vi "synch_mri_to_phys_data_vTriggerRunout.vi"() -> ()   [LabVIEW 2016]
uses:
  <vilib>/DAQmx/read.llb/DAQmx Read (Analog DBL 1Chan 1Samp).vi
  <vilib>/DAQmx/read.llb/DAQmx Read (Digital Bool 1Line 1Point).vi
  <vilib>/DAQmx/create/channels.llb/DAQmx Create Channel (DI-Digital Input).vi
  <vilib>/Instr/_visa.llb/VISA Configure Serial Port (Instr).vi
  <vilib>/DAQmx/create/channels.llb/DAQmx Create Channel (AI-Voltage-Basic).vi
  <vilib>/DAQmx/configure/timing.llb/DAQmx Timing (Sample Clock).vi
  <vilib>/DAQmx/miscellaneous.llb/DAQmx Fill In Error Info.vi
  <vilib>/Utility/file.llb/Write Delimited Spreadsheet (DBL).vi
panel:
  out "appended array":dbl[][](array[numeric])
  out "read buffer":string
  in  "stop":bool
  out "% SpO2":dbl[](graph)
  in  "SpO2 line":tag="MRITrig/ai0"
  out "Inspiration/Expiration":i16[](graph)
  out "Temp":dbl
  out "End":bool
  in  "TEST RUN":bool
  out "Temp (deg C)":dbl(slide) scale=0.0..40.0
  out "% CO_2":dbl format="%0.2f"
  out "% CO2":dbl[](graph)
  out "read byte count":u32=15
  out "write byte count":u32=8
  in  "\"Get Temperature\" command":string="\u0006ùGVT\u0001ð>"
  in  "file path (dialog if empty)":path=path "C:/Users/glihaug/Documents/Project 2/dc/dc171013_scan14_physdata.txt"
  in  "Sampling Rate":dbl=1000.0 format="%0.2f"
  in  "Mechanical Ventilator":tag="MRITrig/port0/line2"
  in  "CO2 line":tag="Dev0/ai1"
  in  "Dummy Ct":dbl=8.0
  out "Trigger Ct":dbl
  in  "COM Port":refnum<visa-resource-name>="COM5"
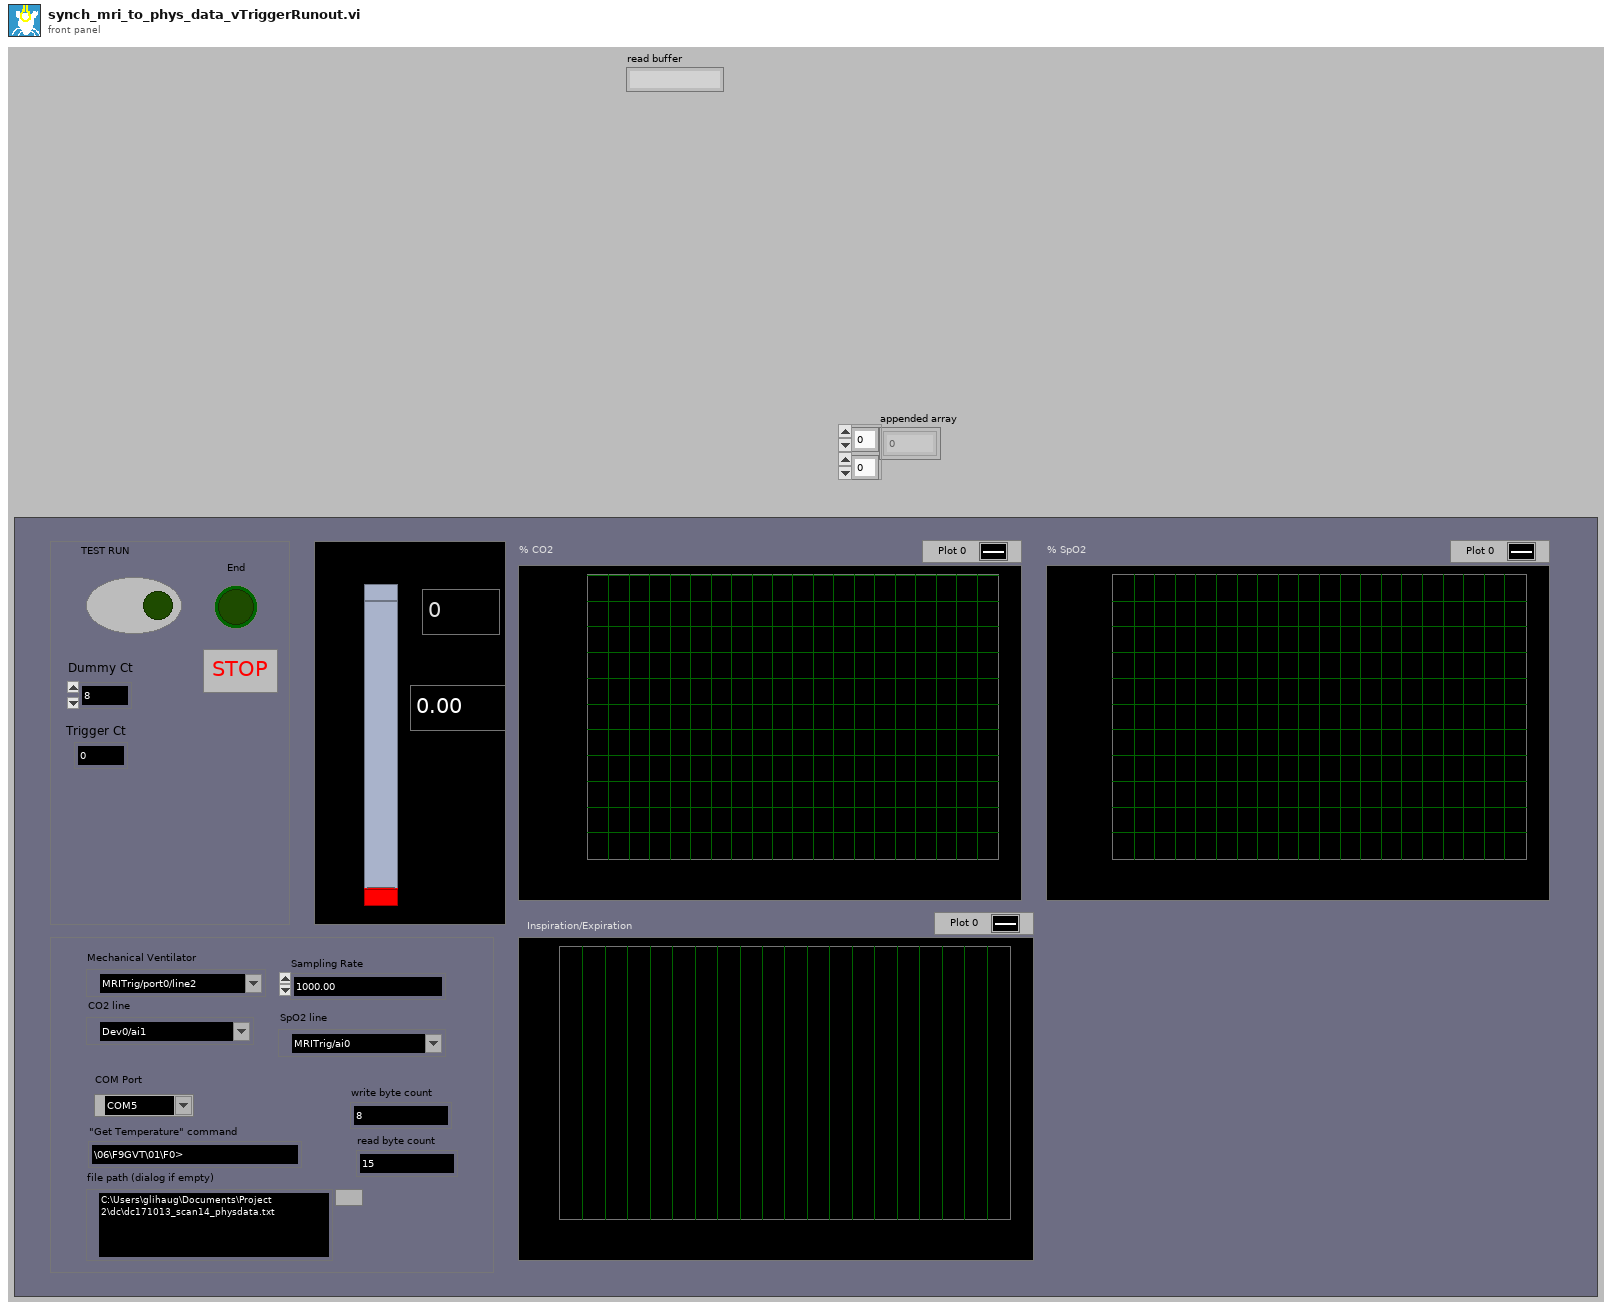
[diagram p1: front panel]
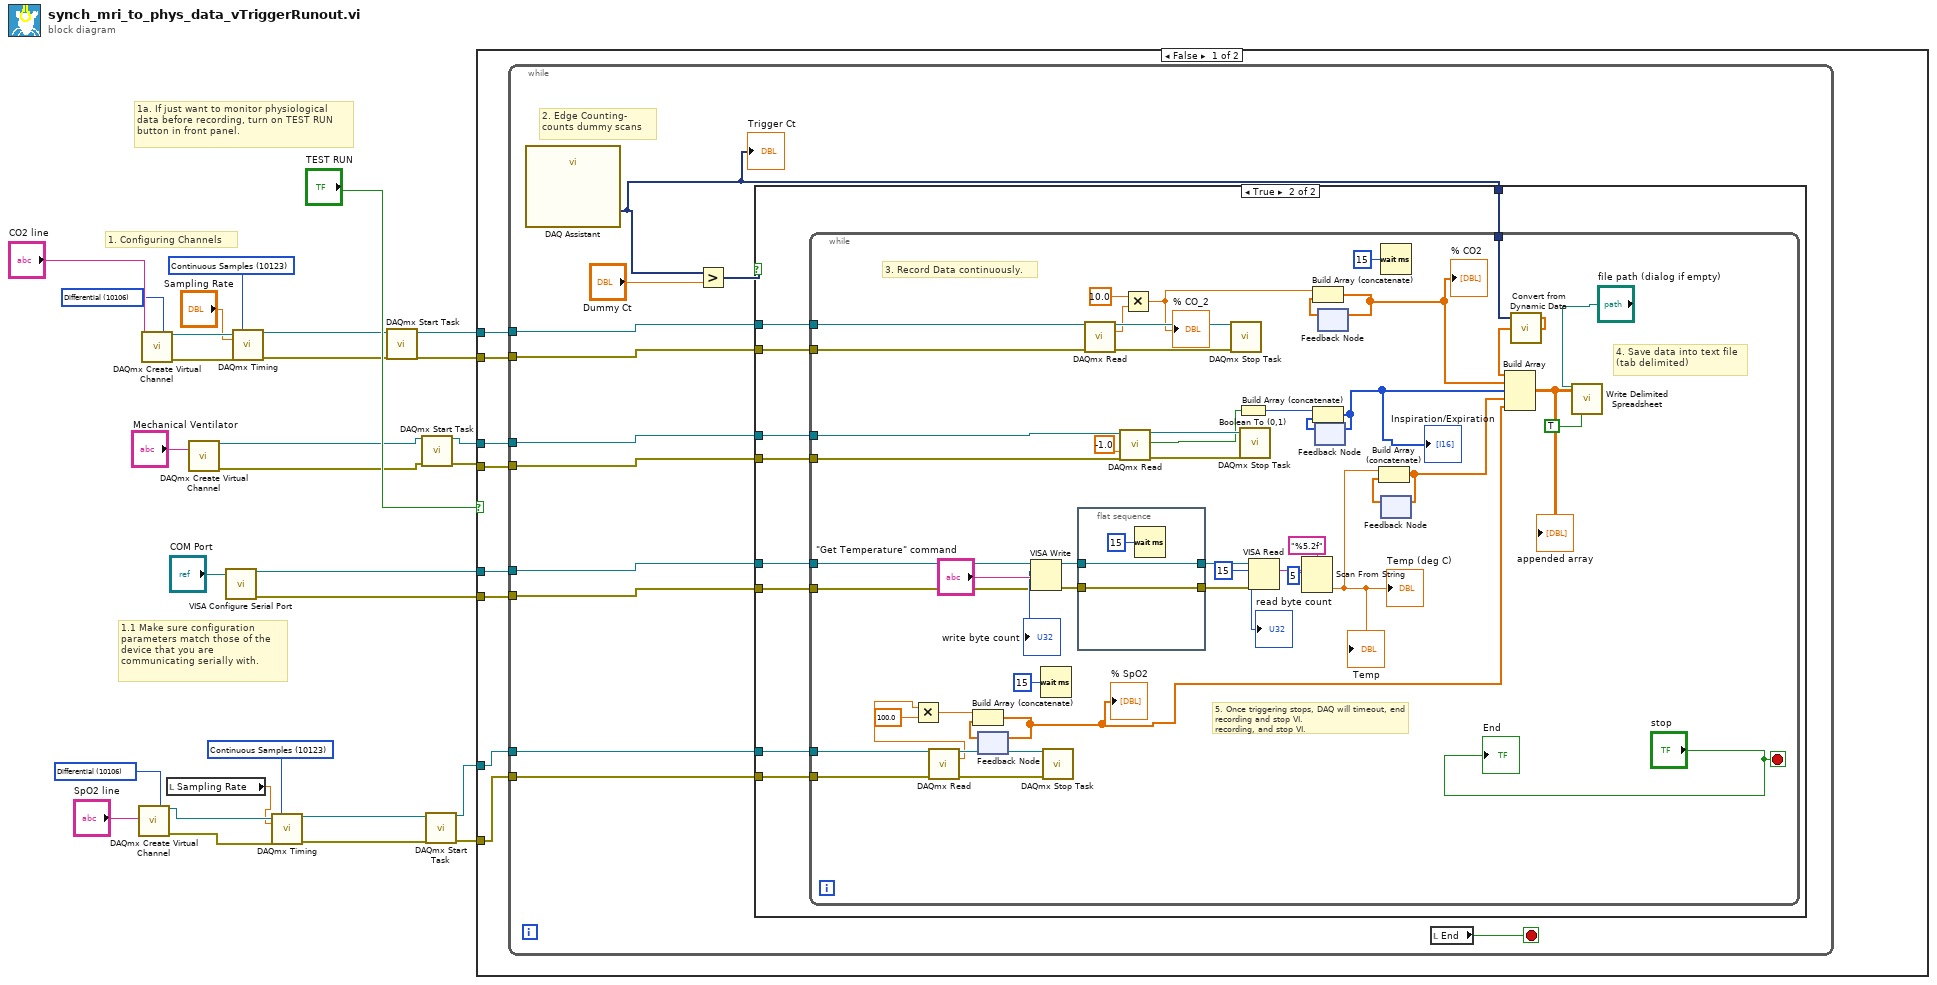
[diagram p0: block diagram]
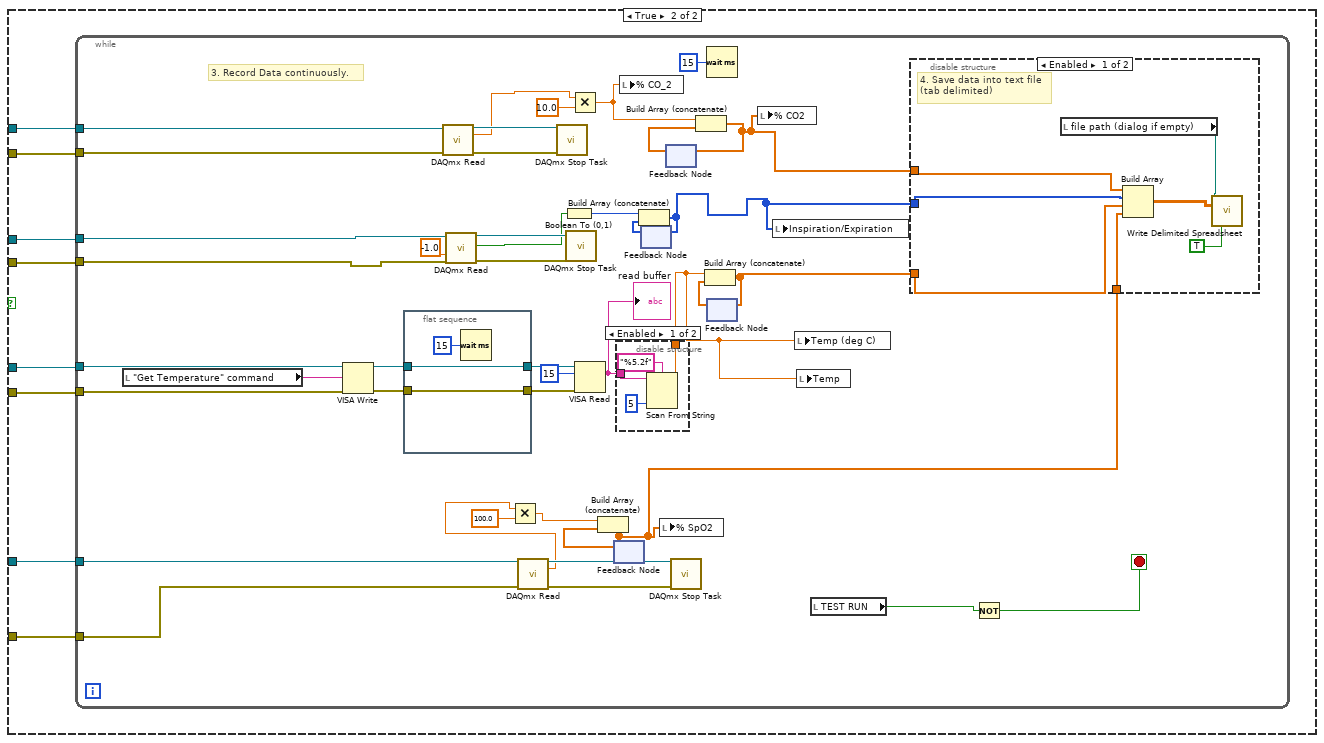
[diagram p3: hidden frame]
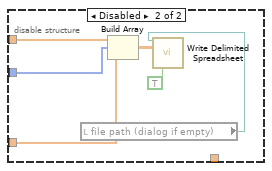
[diagram p5: hidden frame]
diagram:
  w8 = 10123 items=["Finite Samples"=10178, "Continuous Samples"=10123, "Hardware Timed Single Point"=12522] ("sample mode")
  w9 = 10106 items=["Default"=-1, "RSE"=10083, "NRSE"=10078, "Differential"=10106, "Pseudodifferential"=12529] ("input terminal configuration")
  w10 = 10106 items=["Default"=-1, "RSE"=10083, "NRSE"=10078, "Differential"=10106, "Pseudodifferential"=12529] ("input terminal configuration")
  w25 = 10123 items=["Finite Samples"=10178, "Continuous Samples"=10123, "Hardware Timed Single Point"=12522] ("sample mode")
  # "1a. If just want to monitor physiological\ndata before recording, turn on TEST RUN\nbutton in front panel."
  # "1.1 Make sure configuration\nparameters match those of the \ndevice that you are \ncommunicating serially with."
  # "1. Configuring Channels"
  n1 = call-poly <vilib>:"DAQmx Create Virtual Channel.vi"("input terminal configuration"=w9, "physical channels"="SpO2 line") -> ("task out"=w5:refnum<k21>, "error out"=w4:errorcluster)  [unwired: 12 in]
  n2 = call-poly <vilib>:"DAQmx Create Virtual Channel.vi"("input terminal configuration"=w10, "physical channels"="CO2 line") -> ("task out"=w28:refnum<k21>, "error out"=w27:errorcluster)  [unwired: 12 in]
  n3 = local read "Sampling Rate"() -> (w3:dbl)
  n4 = call-poly <vilib>:"DAQmx Create Virtual Channel.vi"("lines"="Mechanical Ventilator") -> ("task out"=w12:refnum<k21>, "error out"=w11:errorcluster)  [unwired: 13 in]
  n5 = call-poly "VISA Configure Serial Port"("VISA resource name"="COM Port") -> ("VISA resource name out"=w22:refnum<visa-resource-name>, "error out"=w21:errorcluster)  [unwired: 13 in]
  n6 = call-poly <vilib>:"DAQmx Timing.vi"("task/channels in"=w28, "sample mode"=w25, "rate"="Sampling Rate", "error in"=w27) -> ("task out"=w18:refnum<k21>, "error out"=w17:errorcluster)  [unwired: 10 in]
  n7 = call-poly <vilib>:"DAQmx Timing.vi"("task/channels in"=w5, "sample mode"=w8, "rate"=w3, "error in"=w4) -> ("task out"=w7:refnum<k21>, "error out"=w6:errorcluster)  [unwired: 10 in]
  n8 = call <vilib>:"DAQmx Start Task.vi"("task/channels in"=w18, "error in"=w17) -> ("task out"=w16:refnum<k21>, "error out"=w15:errorcluster)  [unwired: 12 in]
  n9 = call <vilib>:"DAQmx Start Task.vi"("task/channels in"=w12, "error in"=w11) -> ("task out"=w14:refnum<k21>, "error out"=w13:errorcluster)  [unwired: 12 in]
  n10 = call <vilib>:"DAQmx Start Task.vi"("task/channels in"=w7, "error in"=w6) -> ("task out"=w2:refnum<k21>, "error out"=w1:errorcluster)  [unwired: 12 in]
  n11 = case shown="False" "TEST RUN" {
    tunnel: w16 -> [w33 w116]
    tunnel: w15 -> [w32 w115]
    tunnel: w14 -> [w37 w120]
    tunnel: w13 -> [w36 w119]
    tunnel: w22 -> [w35 w118]
    tunnel: w21 -> [w34 w117]
    tunnel: w2 -> [w31 w114]
    tunnel: w1 -> [w30 w113]
    frame False {
      n12 = while {
        tunnel: w33 -> [w48]
        tunnel: w32 -> [w47]
        tunnel: w37 -> [w46]
        tunnel: w36 -> [w45]
        tunnel: w35 -> [w43]
        tunnel: w34 -> [w42]
        tunnel: w31 -> [w39]
        tunnel: w30 -> [w38]
        stop <- w44 stop-if-true
        # "2. Edge Counting-\ncounts dummy scans"
        n13 = call "DAQ Assistant"() -> ("data"=w40:dynamicdata)  [unwired: 16 in, 3 out]
        "Trigger Ct" <- w40
        n14 = Greater?(x=w40, y="Dummy Ct") -> (0:w49:dynamicdata)
        n15 = case shown="True" w49 {
          tunnel: w48 -> [_ w58]
          tunnel: w47 -> [_ w57]
          tunnel: w46 -> [_ w56]
          tunnel: w45 -> [_ w55]
          tunnel: w43 -> [_ w54]
          tunnel: w42 -> [_ w53]
          tunnel: w40 -> [_ w52]
          tunnel: w39 -> [_ w51]
          tunnel: w38 -> [_ w50]
          frame False {
          }
          frame True {
            n16 = while {
              tunnel: w58 -> [w77]
              tunnel: w57 -> [w76]
              tunnel: w56 -> [w75]
              tunnel: w55 -> [w74]
              tunnel: w54 -> [w95]
              tunnel: w53 -> [w94]
              tunnel: w52 -> [w73]
              tunnel: w51 -> [w63]
              tunnel: w50 -> [w62]
              stop <- "stop" stop-if-true
              # "5. Once triggering stops, DAQ will timeout, end recording and stop VI.\nrecording, and stop VI."
              # "4. Save data into text file \n(tab delimited)"
              # "3. Record Data continuously."
              n17 = call-poly <vilib>:"DAQmx Read.vi"("task/channels in"=w63, "error in"=w62) -> ("task out"=w67:refnum<k21>, "data"=w59:dbl, "error out"=w66:errorcluster)  [unwired: 11 in]
              n18 = Multiply(x=w59, y=100.0) -> (x*y=w60:dbl)
              n19 = feedback #1() -> (w64:dbl[])  [unwired: 1 in]
              n20 = Build Array (concatenate)(w60, w64) -> (w78:dbl[])
              "% SpO2" <- w78
              n21 = feedback-in #1(w78) -> ()
              n22 = VISA Write(VISA resource name=w95, write buffer="\"Get Temperature\" command", error in (no error)=w94) -> (VISA resource name out=w101:refnum<visa-resource-name>, return count=→"write byte count":u32, error out=w99:errorcluster)
              n23 = Wait (ms)(milliseconds to wait=u32 15) -> ()  [unwired: 1 out]
              n24 = call <vilib>:"DAQmx Stop Task.vi"("task/channels in"=w67, "error in"=w66) -> ()  [unwired: 12 in, 2 out]
              n25 = flat-sequence {
                tunnel: [w112] -> w100
                tunnel: w101 -> [w112]
                tunnel: w99 -> [w111]
                tunnel: [w111] -> w98
                frame #0 {
                  n26 = Wait (ms)(milliseconds to wait=u32 15) -> ()  [unwired: 1 out]
                }
              }
              n27 = call-poly <vilib>:"DAQmx Read.vi"("task/channels in"=w77, "error in"=w76) -> ("task out"=w106:refnum<k21>, "data"=w70:dbl, "error out"=w105:errorcluster)  [unwired: 11 in]
              n28 = call-poly <vilib>:"DAQmx Read.vi"("task/channels in"=w75, "timeout"=-1.0, "error in"=w74) -> ("task out"=w108:refnum<k21>, "data"=w93:bool, "error out"=w107:errorcluster)  [unwired: 10 in]
              n29 = Multiply(x=10.0, y=w70) -> (x*y=w68:dbl)
              "% CO_2" <- w68
              n30 = call <vilib>:"DAQmx Stop Task.vi"("task/channels in"=w106, "error in"=w105) -> ()  [unwired: 12 in, 2 out]
              n31 = Boolean To (0,1)(Boolean=w93) -> (0, 1=w90:i16)
              n32 = call <vilib>:"DAQmx Stop Task.vi"("task/channels in"=w108, "error in"=w107) -> ()  [unwired: 12 in, 2 out]
              n33 = VISA Read(VISA resource name=w100, byte count=u32 15, error in (no error)=w98) -> (read buffer=w83:string, return count=→"read byte count":u32)  [unwired: 2 out]
              n34 = Scan From String(format string="%5.2f", input string=w83, initial scan location=u32 5) -> (output 1=w82:dbl)  [unwired: 2 in, 3 out]
              "Temp (deg C)" <- w82
              "Temp" <- w82
              n35 = feedback #2() -> (w89:i16[])  [unwired: 1 in]
              n36 = Build Array (concatenate)(w90, w89) -> (w81:i16[])
              "Inspiration/Expiration" <- w81
              n37 = feedback-in #2(w81) -> ()
              n38 = feedback #3() -> (w92:dbl[])  [unwired: 1 in]
              n39 = Build Array (concatenate)(w68, w92) -> (w80:dbl[])
              "% CO2" <- w80
              n40 = feedback-in #3(w80) -> ()
              n41 = Wait (ms)(milliseconds to wait=u32 15) -> ()  [unwired: 1 out]
              n42 = feedback #4() -> (w88:dbl[])  [unwired: 1 in]
              n43 = Build Array (concatenate)(w82, w88) -> (w87:dbl[])
              n44 = feedback-in #4(w87) -> ()
              n45 = call "Convert from Dynamic Data"("Dynamic Data Type"=w73) -> ("Array"=w72:dbl[])  [unwired: 3 in]
              n46 = Build Array(w72, w80, w81, w87, w78) -> (w71:dbl[][])
              "appended array" <- w71
              n47 = call-poly <vilib>:"Write Delimited Spreadsheet.vi"("file path (dialog if empty)"="file path (dialog if empty)", "2D data"=w71, "transpose? (no:F)"=TRUE) -> ()  [unwired: 11 in, 2 out]
              "End" <- "stop"
            }
          }
        }
        n48 = local read "End"() -> (w44:bool)
      }
    }
    frame True {
      n49 = while {
        tunnel: w115 -> [w139]
        tunnel: w120 -> [w138]
        tunnel: w119 -> [w137]
        tunnel: w118 -> [w144]
        tunnel: w117 -> [w151]
        tunnel: w116 -> [w136]
        tunnel: w114 -> [w126]
        tunnel: w113 -> [w125]
        stop <- w141 stop-if-true
        # "3. Record Data continuously."
        n50 = local read "\"Get Temperature\" command"() -> (w143:string)
        n51 = VISA Write(VISA resource name=w144, write buffer=w143, error in (no error)=w151) -> (VISA resource name out=w155:refnum<visa-resource-name>, error out=w153:errorcluster)  [unwired: 1 out]
        n52 = flat-sequence {
          tunnel: [w182] -> w154
          tunnel: w155 -> [w182]
          tunnel: w153 -> [w181]
          tunnel: [w181] -> w152
          frame #0 {
            n53 = Wait (ms)(milliseconds to wait=u32 15) -> ()  [unwired: 1 out]
          }
        }
        n54 = call-poly <vilib>:"DAQmx Read.vi"("task/channels in"=w136, "error in"=w139) -> ("task out"=w159:refnum<k21>, "data"=w133:dbl, "error out"=w158:errorcluster)  [unwired: 11 in]
        n55 = call-poly <vilib>:"DAQmx Read.vi"("task/channels in"=w138, "timeout"=-1.0, "error in"=w137) -> ("task out"=w161:refnum<k21>, "data"=w150:bool, "error out"=w160:errorcluster)  [unwired: 10 in]
        n56 = call-poly <vilib>:"DAQmx Read.vi"("task/channels in"=w126, "error in"=w125) -> ("task out"=w129:refnum<k21>, "data"=w122:dbl, "error out"=w128:errorcluster)  [unwired: 11 in]
        n57 = Multiply(x=w122, y=100.0) -> (x*y=w123:dbl)
        n58 = call <vilib>:"DAQmx Stop Task.vi"("task/channels in"=w159, "error in"=w158) -> ()  [unwired: 12 in, 2 out]
        n59 = Boolean To (0,1)(Boolean=w150) -> (0, 1=w149:i16)
        n60 = call <vilib>:"DAQmx Stop Task.vi"("task/channels in"=w161, "error in"=w160) -> ()  [unwired: 12 in, 2 out]
        n61 = Multiply(x=w133, y=10.0) -> (x*y=w132:dbl)
        n62 = VISA Read(VISA resource name=w154, byte count=u32 15, error in (no error)=w152) -> (read buffer=w145:string)  [unwired: 3 out]
        "read buffer" <- w145
        n63 = feedback #5() -> (w127:dbl[])  [unwired: 1 in]
        n64 = Build Array (concatenate)(w123, w127) -> (w121:dbl[])
        n65 = feedback-in #5(w121) -> ()
        n66 = disable-structure shown="Enabled" {
          disable-tunnel: w145 -> [w164 _]
          disable-tunnel: [w163 _] -> w140
          frame Enabled {
            n67 = Scan From String(format string="%5.2f", input string=w164, initial scan location=u32 5) -> (output 1=w163:dbl)  [unwired: 2 in, 3 out]
          }
          frame Disabled {
          }
        }
        n68 = local write "% CO_2"(w132) -> ()
        n69 = feedback #6() -> (w148:i16[])  [unwired: 1 in]
        n70 = Build Array (concatenate)(w149, w148) -> (w135:i16[])
        n71 = feedback-in #6(w135) -> ()
        n72 = local write "% SpO2"(w121) -> ()
        n73 = feedback #7() -> (w131:dbl[])  [unwired: 1 in]
        n74 = call <vilib>:"DAQmx Stop Task.vi"("task/channels in"=w129, "error in"=w128) -> ()  [unwired: 12 in, 2 out]
        n75 = Build Array (concatenate)(w132, w131) -> (w130:dbl[])
        n76 = feedback-in #7(w130) -> ()
        n77 = Wait (ms)(milliseconds to wait=u32 15) -> ()  [unwired: 1 out]
        n78 = feedback #8() -> (w147:dbl[])  [unwired: 1 in]
        n79 = Build Array (concatenate)(w140, w147) -> (w146:dbl[])
        n80 = feedback-in #8(w146) -> ()
        n81 = local write "% CO2"(w130) -> ()
        n82 = local write "Inspiration/Expiration"(w135) -> ()
        n83 = local write "Temp (deg C)"(w140) -> ()
        n84 = local write "Temp"(w140) -> ()
        n85 = local read "TEST RUN"() -> (w142:bool)
        n86 = disable-structure shown="Enabled" {
          disable-tunnel: w146 -> [w173 w177]
          disable-tunnel: w130 -> [w172 w176]
          disable-tunnel: w135 -> [w171 w175]
          disable-tunnel: w121 -> [w167 _]
          frame Enabled {
            # "4. Save data into text file \n(tab delimited)"
            n87 = local read "file path (dialog if empty)"() -> (w169:path)
            n88 = Build Array(w172, w171, w173, w167) -> (w170:dbl[][])
            n89 = call-poly <vilib>:"Write Delimited Spreadsheet.vi"("file path (dialog if empty)"=w169, "2D data"=w170, "transpose? (no:F)"=TRUE) -> ()  [unwired: 11 in, 2 out]
          }
          frame Disabled {
            n90 = local read "file path (dialog if empty)"() -> (w174:path)
            n91 = Build Array(w176, w175, w177) -> (w178:dbl[][])
            n92 = call-poly <vilib>:"Write Delimited Spreadsheet.vi"("file path (dialog if empty)"=w174, "2D data"=w178, "transpose? (no:F)"=TRUE) -> ()  [unwired: 11 in, 2 out]
          }
        }
        n93 = Not(x=w142) -> (.not. x?=w141:bool)
      }
    }
  }
